vi "Get Plugin Configuration.vi"(8 "error in (no error)":errorcluster, 11 "Component Configuration in":refnum<class "Core Component Configurations.lvclass">) -> (0 "error out":errorcluster, 2 "Plugin Configuration":refnum<class "Configuration.lvclass">, 3 "Component Configuration out":refnum<class "Core Component Configurations.lvclass">)   [LabVIEW 2021, in "DSF Core.lvlib" / "Core Component Configurations.lvclass"]
uses:
  Core Component Configurations.lvclass
  Configuration/Configuration.lvclass
  Configuration/Core/Plugin/Plugin Configuration.lvclass
  C:/dev/git/custom-devices/niveristand-data-sharing-framework-custom-device/Source/Core/Classes/Configuration/Configuration.lvclass
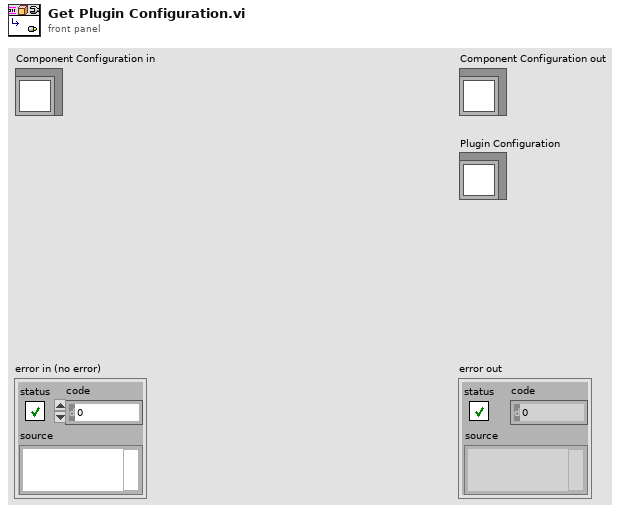
[diagram p1: front panel]
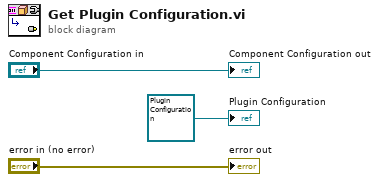
[diagram p0: block diagram]
diagram:
  "error out" <- "error in (no error)"
  "Component Configuration out" <- "Component Configuration in"
  "Plugin Configuration" <- refnum<class "Plugin Configuration.lvclass"> refnum ("DSF Core.lvlib:Plugin Configuration.lvclass")
